vi "double_exponential_smoothing _2.vi"(1 "x":dbl, 2 "alpha":dbl) -> (0 "dema":dbl)   [LabVIEW 2019]
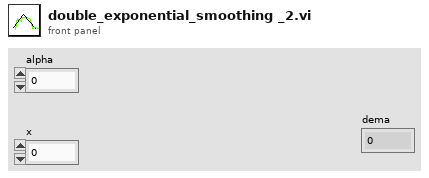
[diagram p1: front panel]
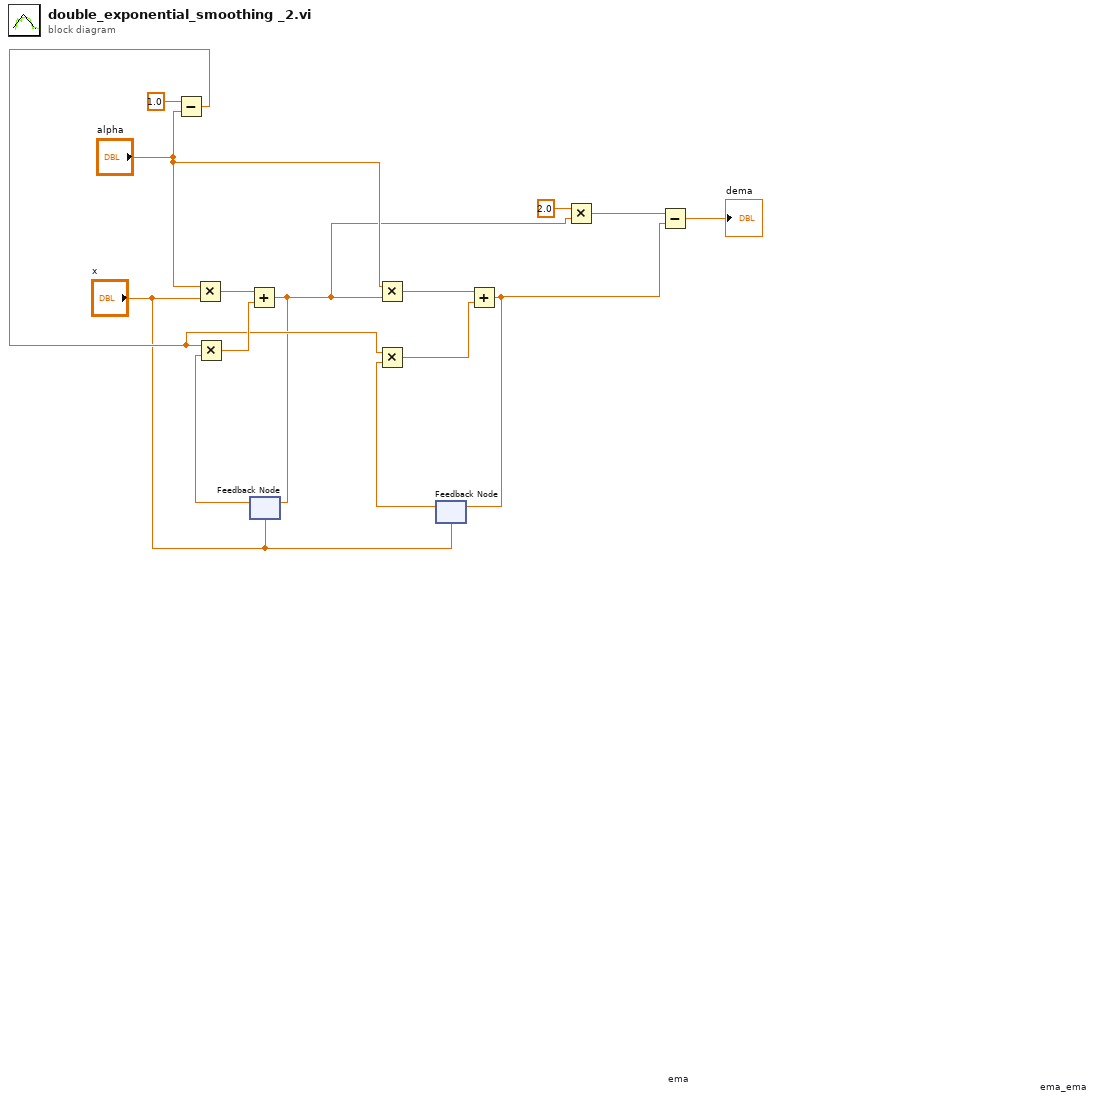
[diagram p0: block diagram]
diagram:
  n1 = Subtract(x=1.0, y="alpha") -> (x-y=w8:dbl)
  n2 = Multiply(x="alpha", y="x") -> (x*y=w14:dbl)
  n3 = feedback #1 "ema"("x") -> (w13:dbl)
  n4 = Multiply(x=w8, y=w13) -> (x*y=w12:dbl)
  n5 = Add(x=w14, y=w12) -> (x+y=w5:dbl)
  n6 = feedback-in #1(w5) -> ()
  n7 = Multiply(x="alpha", y=w5) -> (x*y=w10:dbl)
  n8 = feedback #2 "ema_ema"("x") -> (w9:dbl)
  n9 = Multiply(x=w8, y=w9) -> (x*y=w7:dbl)
  n10 = Add(x=w10, y=w7) -> (x+y=w3:dbl)
  n11 = feedback-in #2(w3) -> ()
  n12 = Multiply(x=2.0, y=w5) -> (x*y=w4:dbl)
  n13 = Subtract(x=w4, y=w3) -> (x-y=→"dema":dbl)
